vi "Client - Error Handler.vi"(7 "Component":string="Archive", 8 "error in (no error)":errorcluster, 11 "Message Queue":refnum<queue>) -> (0 "error out":errorcluster)   [LabVIEW 2024]
doc: "Handles errors in the client."
uses:
  Support/Shared/Message Queue/Message Cluster.ctl
  Support/Shared/Message Queue.lvlib
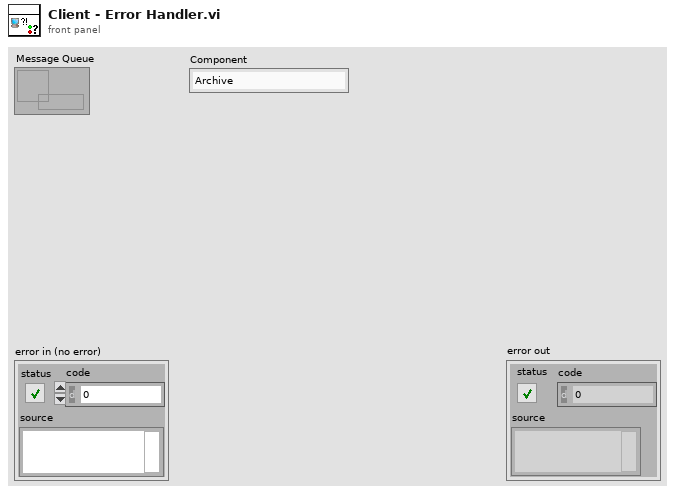
[diagram p1: front panel]
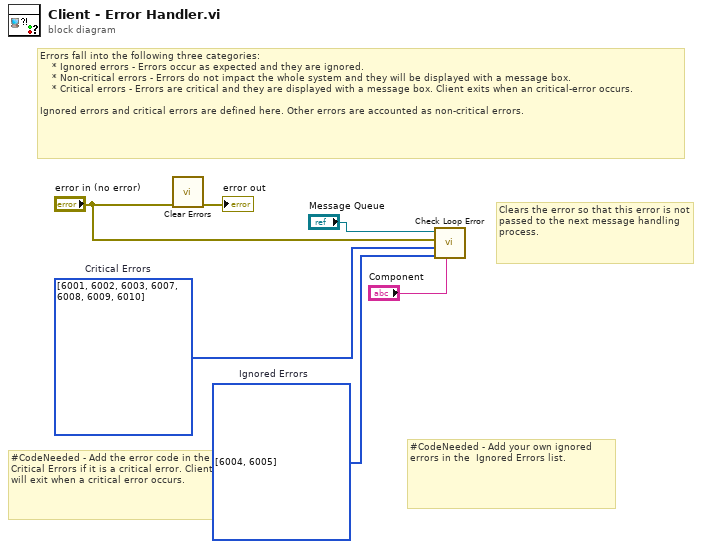
[diagram p0: block diagram]
diagram:
  w2 = i32[] [6004, 6005]  # Ignored Errors
  w6 = i32[] [6001, 6002, 6003, 6007, 6008, 6009, 6010]  # Critical Errors
  # "#CodeNeeded - Add your own ignored errors in the  Ignored Errors list."
  # "#CodeNeeded - Add the error code in the Critical Errors if it is a critical error. Client will exit when a critical error occurs."
  # "Errors fall into the following three categories:\t \n  \t\t* Ignored errors - Errors occur as expected and they are ignored. \n  \t\t* Non-critical errors - Errors do not impact the whole system and they will be displayed with a message box.\n\t\t  * Critical errors - Errors are critical and they are displayed with a message box. Client exits when an critical-error occurs.\n\nIgnored errors and critical errors are defined here. Other errors are accounted as non-critical errors."
  # "Clears the error so that this error is not passed to the next message handling process."
  n1 = call <vilib>:"Clear Errors.vi"("error in (no error)"="error in (no error)") -> ("error out"=→"error out":errorcluster)  [unwired: 5 in, 1 out]
  n2 = call "Check Loop Error.vi"("Component"="Component", "Ignored Errors"=w2, "Critical Errors"=w6, "Error to Handle"="error in (no error)", "Message Queue"="Message Queue") -> ()  [unwired: 7 in]
